vi "digital.vi"(10 "DIGITAL":T1={"Puertos Digital"=[], "Lineas Digital"=[], "Frecuencia Muestreo"=1000, "Puerto/Linea"=FALSE}, 11 "Adquisicion tiempo":i32) -> ()   [LabVIEW 2020, in "Settings.lvlib"]
uses:
  Settings.lvlib
  Acquisition/cluster digital.ctl
  <vilib>/drjdpowell/SQLite Library/SQL Connection/Open (path).vi
  <vilib>/drjdpowell/SQLite Library/SQL Connection/Open (string).vi
  <vilib>/AdvancedString/Path To Command Line String.vi
  <vilib>/drjdpowell/SQLite Library/SQL Connection/Execute SQL (No results).vi
  <vilib>/drjdpowell/SQLite Library/SQL Connection/Connection.lvclass
  <vilib>/drjdpowell/SQLite Library/SQLite.lvlib
  Acquisition/CONTROLS.lvlib
panel:
  out "error out":errorcluster
  in  "error in (no error)":errorcluster
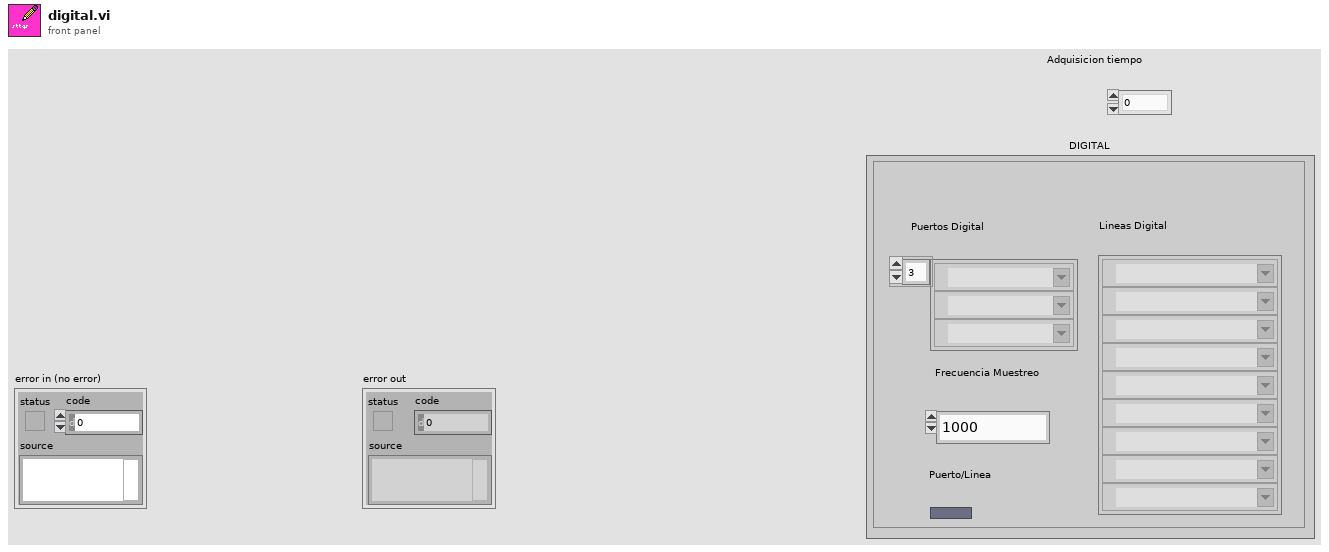
[diagram p1: front panel]
types:
  T1 = typedef "Acquisition.lvlib/CONTROLS.lvlib/cluster digital.ctl" = cluster{"Puertos Digital":tag[], "Lineas Digital":tag[], "Frecuencia Muestreo":u32, "Puerto/Linea":bool}
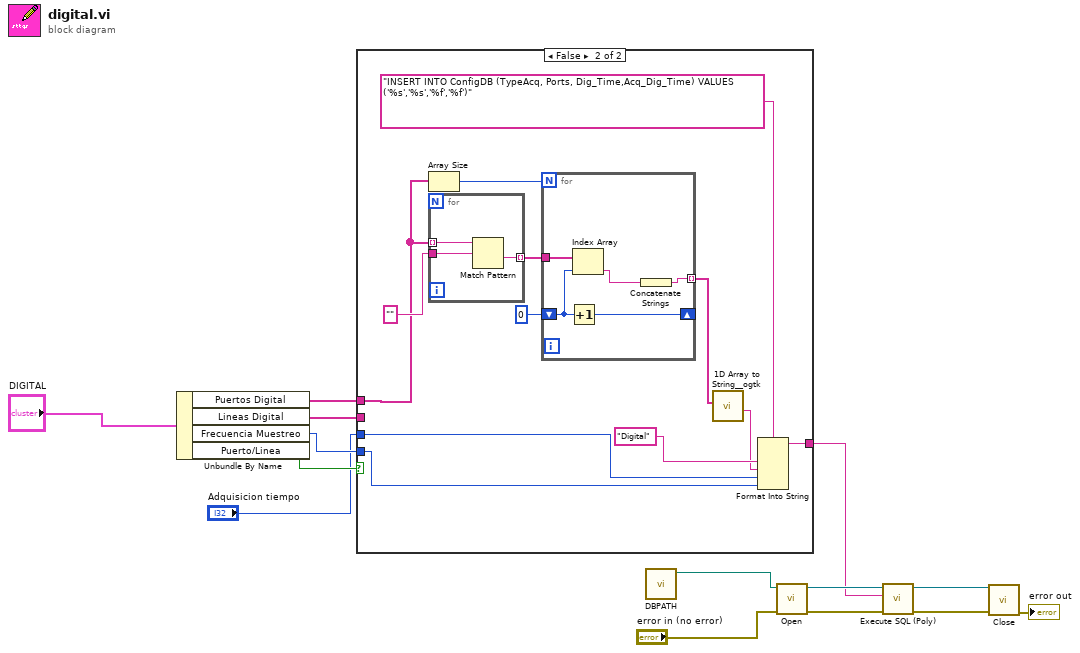
[diagram p0: block diagram]
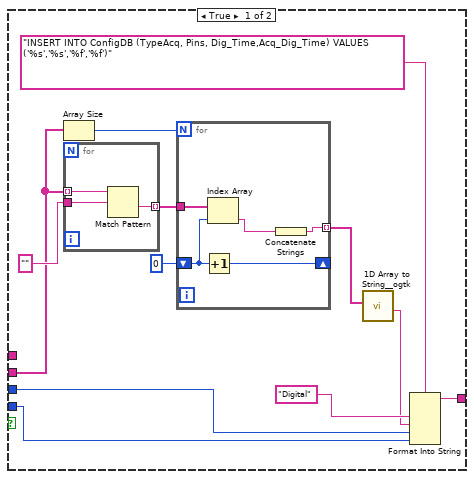
[diagram p2: hidden frame]
diagram:
  n1 = Unbundle By Name("DIGITAL") -> ("Puertos Digital"=w8:tag[], "Lineas Digital"=w7:tag[], "Frecuencia Muestreo"=w2:u32, "Puerto/Linea"=w3:bool)
  n2 = case shown="False" w3 {
    tunnel: w8 -> [_ w37]
    tunnel: w7 -> [w20 _]
    tunnel: "Adquisicion tiempo" -> [w18 w35]
    tunnel: w2 -> [w17 w44]
    tunnel: [w19 w45] -> w6
    frame True {
      n3 = Array Size(array=w20) -> (size(s)=w24:i32)
      n4 = for {
        tunnel: w20 -> [w29] mode=indexing
        tunnel: [w28] -> w23 mode=indexing
        tunnel: "" ("regular expression") -> [w27]
        n5 = Match Pattern(string=w29, regular expression=w27) -> (after substring=w28:string)  [unwired: 1 in, 3 out]
      }
      n6 = for {
        N: w24 -> [_]
        shift-right: [w32] -> _
        shift-left: 0 -> [w33]
        tunnel: w23 -> [w34]
        tunnel: [w30] -> w25 mode=indexing
        n7 = Increment(x=w33) -> (x+1=w32:i32)
        n8 = Index Array(array=w34, index=w33) -> (element=w31:string)
        n9 = Concatenate Strings(w31) -> (w30:string)
      }
      n10 = call <userlib>:"1D Array to String__ogtk.vi"("Array of Strings"=w25) -> ("delimited string"=w15:string)  [unwired: 10 in]
      n11 = Format Into String(format string="INSERT INTO ConfigDB (TypeAcq, Pins, Dig_Time,Acq_Dig_Time) VALUES ('%s','%s','%f','%f')", "Digital" ("input 1"), w15, w18, w17) -> (resulting string=w19:string)  [unwired: 2 in, 1 out]
    }
    frame False {
      n12 = Array Size(array=w37) -> (size(s)=w41:i32)
      n13 = for {
        tunnel: w37 -> [w49] mode=indexing
        tunnel: [w48] -> w40 mode=indexing
        tunnel: "" ("regular expression") -> [w47]
        n14 = Match Pattern(string=w49, regular expression=w47) -> (after substring=w48:string)  [unwired: 1 in, 3 out]
      }
      n15 = for {
        N: w41 -> [_]
        shift-right: [w52] -> _
        shift-left: 0 -> [w53]
        tunnel: w40 -> [w54]
        tunnel: [w50] -> w42 mode=indexing
        n16 = Increment(x=w53) -> (x+1=w52:i32)
        n17 = Index Array(array=w54, index=w53) -> (element=w51:string)
        n18 = Concatenate Strings(w51) -> (w50:string)
      }
      n19 = call <userlib>:"1D Array to String__ogtk.vi"("Array of Strings"=w42) -> ("delimited string"=w36:string)  [unwired: 10 in]
      n20 = Format Into String(format string="INSERT INTO ConfigDB (TypeAcq, Ports, Dig_Time,Acq_Dig_Time) VALUES ('%s','%s','%f','%f')", "Digital" ("input 1"), w36, w35, w44) -> (resulting string=w45:string)  [unwired: 2 in, 1 out]
    }
  }
  n21 = call "DBPATH.vi"() -> ("appended path"=w5:path)  [unwired: 11 in]
  n22 = call-poly <vilib>:"Open.vi"("error in (no error)"="error in (no error)", "db file"=w5) -> ("error out"=w14:errorcluster, "SQLite Connection"=w12:refnum<class "Connection.lvclass">)  [unwired: 8 in]
  n23 = call-poly <vilib>:"Execute SQL (Poly).vi"("error in (no error)"=w14, "SQL"=w6, "SQLite Connection in"=w12) -> ("error out"=w13:errorcluster, "SQLite Connection"=w11:refnum<class "Connection.lvclass">)  [unwired: 7 in]
  n24 = call-dynamic "Close.vi"("error in (no error)"=w13, "SQLite Connection in"=w11) -> ("error out"=→"error out":errorcluster)  [unwired: 9 in]
